vi "Extract Unique IDs from Stats.vi"(9 "Stats":string[][](array[string]), 11 "Data":string[][](array[string])) -> (1 "Stats with IDs":string[][](array[string]), 3 "Data with IDs":string[][](array[string]))   [LabVIEW 2013]
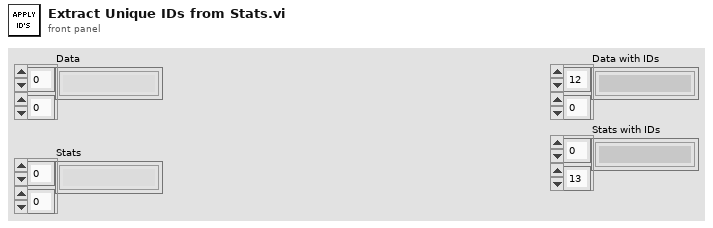
[diagram p1: front panel]
types:
  T1 = cluster{"disabled index (col)":i32, string[], string[]}
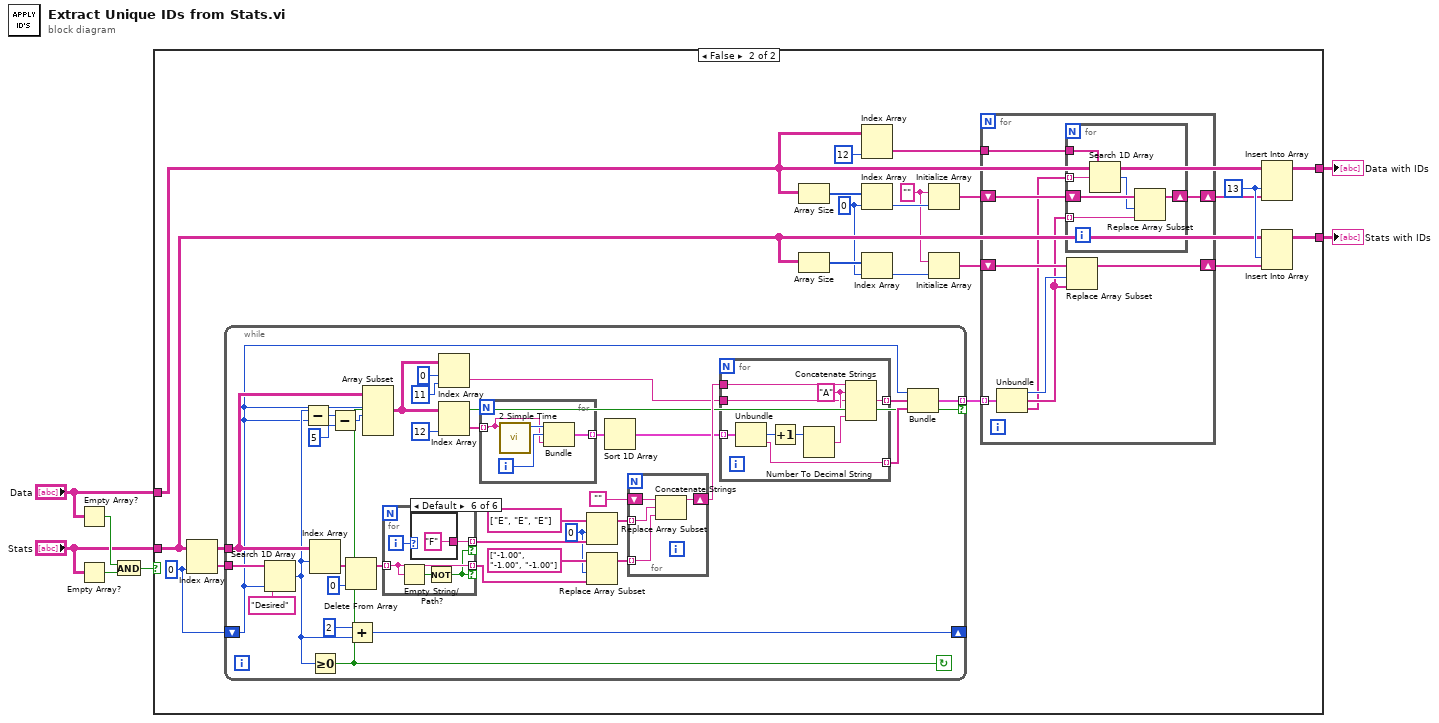
[diagram p0: block diagram]
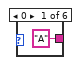
[diagram p3: hidden frame]
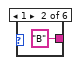
[diagram p4: hidden frame]
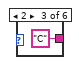
[diagram p5: hidden frame]
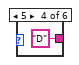
[diagram p6: hidden frame]
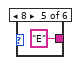
[diagram p7: hidden frame]
diagram:
  n1 = Empty Array?(array="Data") -> (empty?=w7:bool)
  n2 = Empty Array?(array="Stats") -> (empty?=w6:bool)
  n3 = And(x=w7, y=w6) -> (x .and. y?=w5:bool)
  n4 = case shown="False" w5 {
    tunnel: "Data" -> [w9 w12]
    tunnel: "Stats" -> [w8 w25]
    tunnel: [w9 w10] -> w2
    tunnel: [w8 w13] -> w1
    frame True {
    }
    frame False {
      w18 = 0 ("index")
      w20 = ""
      w27 = 13 ("disabled index (col)")
      w28 = 0 ("disabled index (col)")
      n5 = Index Array(array=w25, index (col)=w28) -> (element=w29:string[])  [unwired: 1 in]
      n6 = while {
        tunnel: w29 -> [w78]
        tunnel: w25 -> [w63]
        shift-right: [w75] -> _
        shift-left: w28 -> [w52]
        tunnel: [w49] -> w26 mode=indexing if=w48
        stop <- w48 continue-if-true
        w68 = 0 ("index")
        n7 = Search 1D Array(1D array=w78, element="Desired", start index (0)=w52) -> (index of element=w62:i32)
        n8 = Subtract(x=w62, y=w52) -> (x-y=w47:i32)
        n9 = Index Array(array=w63, index (row)=w62) -> (element=w74:string[])  [unwired: 1 in]
        n10 = Greater Or Equal To 0?(x=w62) -> (x >= 0?=w48:bool)
        n11 = Subtract(x=w47, y=5) -> (x-y=w46:i32)
        n12 = Delete From Array(array=w74, index=0) -> (array with subset deleted=w72:string[])  [unwired: 1 in, 1 out]
        n13 = Add(x=2, y=w62) -> (x+y=w75:i32)
        n14 = Array Subset(array=w63, index (row)=w52, length (row)=w46) -> (w58:string[][])  [unwired: 2 in]
        n15 = for {
          tunnel: w72 -> [w100] mode=indexing
          tunnel: [w96] -> w70 mode=indexing if=w98
          tunnel: [w100] -> w67 mode=indexing if=w98
          i -> [w97]
          n16 = Empty String/Path?(string/path=w100) -> (empty?=w99:bool)
          n17 = case shown="Default" w97 {
            tunnel: ["A" "B" "C" "D" "E" "F"] -> w96
            frame 0 {
            }
            frame 1 {
            }
            frame 2 {
            }
            frame 5 {
            }
            frame 8 {
            }
            frame Default {
            }
          }
          n18 = Not(x=w99) -> (.not. x?=w98:bool)
        }
        n19 = Index Array(array=w58, index (row)=0, index (col)=11 ("disabled index (col)")) -> (element=w53:string)
        n20 = Index Array(array=w58, index (col)=12 ("disabled index (col)")) -> (element=w60:string[])  [unwired: 1 in]
        n21 = for {
          tunnel: w60 -> [w88] mode=indexing
          tunnel: [w89] -> w59 mode=indexing
          i -> [w90]
          n22 = call "2 Simple Time.vi"("Timestamp"=w88) -> ("Simple Time"=w91:i64)  [unwired: 9 in, 1 out]
          n23 = Bundle("Simple Time"=w91, w90, w88) -> (w89:cluster{"Simple Time":i64, i32, string})  [unwired: 1 in]
        }
        n24 = Replace Array Subset(array=string[] ["E", "E", "E"], new element=w70, index=w68) -> (w66:string[])
        n25 = Replace Array Subset(array=string[] ["-1.00", "-1.00", "-1.00"], new element=w67, index=w68) -> (w65:string[])
        n26 = Sort 1D Array(array=w59) -> (sorted array=w54:cluster{"Simple Time":i64, i32, string}[])
        n27 = for {
          tunnel: w66 -> [w93] mode=indexing
          tunnel: w65 -> [w92] mode=indexing
          shift-right: [w94] -> w55
          shift-left: "" -> [w95]
          n28 = Concatenate Strings(w95, w93, w92) -> (w94:string)
        }
        n29 = for {
          tunnel: w55 -> [w85]
          tunnel: w54 -> [w87] mode=indexing
          tunnel: w53 -> [w83]
          tunnel: [w80] -> w51 mode=indexing
          tunnel: [w79] -> w50 mode=indexing
          w84 = "A" ("string")
          n30 = Unbundle(w87) -> (w86:i32, w79:string)  [unwired: 1 out]
          n31 = Increment(x=w86) -> (x+1=w82:i32)
          n32 = Number To Decimal String(number=w82) -> (decimal integer string=w81:string)  [unwired: 1 in]
          n33 = Concatenate Strings(w85, w84, w83, w84, w81) -> (w80:string)
        }
        n34 = Bundle("disabled index (col)"=w52, w51, w50) -> (w49:T1)  [unwired: 1 in]
      }
      n35 = Array Size(array=w12) -> (size(s)=w24:i32[])
      n36 = Array Size(array=w25) -> (size(s)=w23:i32[])
      n37 = Index Array(array=w12, index (col)=12 ("disabled index (col)")) -> (element=w14:string[])  [unwired: 1 in]
      n38 = Index Array(array=w24, index=w18) -> (element=w22:i32)
      n39 = Index Array(array=w23, index=w18) -> (element=w21:i32)
      n40 = Initialize Array(w20, w22) -> (w19:string[])
      n41 = Initialize Array(w20, w21) -> (w17:string[])
      n42 = for {
        tunnel: w26 -> [w38] mode=indexing
        shift-right: [w30] -> w11
        shift-left: w19 -> [w34]
        shift-right: [w35] -> w16
        shift-left: w17 -> [w37]
        tunnel: w14 -> [w31]
        n43 = Unbundle(w38) -> ("disabled index (col)"=w36:i32, w33:string[], w32:string[])
        n44 = for {
          shift-right: [w41] -> w30
          shift-left: w34 -> [w42]
          tunnel: w33 -> [w39] mode=indexing
          tunnel: w32 -> [w43] mode=indexing
          tunnel: w31 -> [w44]
          n45 = Search 1D Array(1D array=w44, element=w43) -> (index of element=w40:i32)  [unwired: 1 in]
          n46 = Replace Array Subset(array=w42, new element=w39, index=w40) -> (w41:string[])
        }
        n47 = Replace Array Subset(array=w37, new element=w33, index=w36) -> (w35:string[])
      }
      n48 = Insert Into Array(array=w12, index (col)=w27, new element=w11) -> (w10:string[][])  [unwired: 1 in]
      n49 = Insert Into Array(array=w25, index (col)=w27, new element=w16) -> (w13:string[][])  [unwired: 1 in]
    }
  }
  "Data with IDs" <- w2
  "Stats with IDs" <- w1
